vi "Handle Sub Device.vi"(0 "Stand in":refnum<class "Stand.lvclass">, 11 "error in (no error)":errorcluster) -> (4 "Stand out":refnum<class "Stand.lvclass">, 14 "dt PMG":u32, 15 "error out":errorcluster)   [LabVIEW 2019, in "Stand.lvclass"]
uses:
  Stand.lvclass
  Stand.lvclass/Stand.ctl
  PM_Group_class/PM_Group.lvclass/PM_Group.ctl
  PM_Group_class/HandleCmd.vi
  PM_Group_class/private/Handle M24.vi
  PM_Group_class/private/Handle M12.vi
  PM_Group_class/private/Handle M21.vi
  Engine_1DO_2DI_class/UpdateEngine.vi
  PM_Group_class/PM_Group.lvclass
  Valve_2DO_2DI_class/Valve_2DO_2DI.lvclass
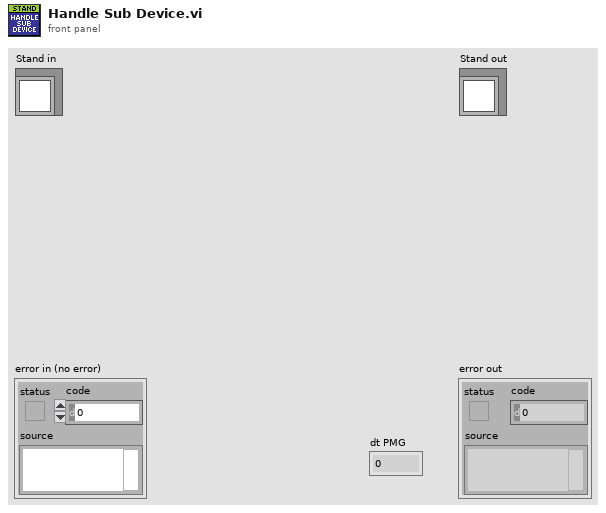
[diagram p1: front panel]
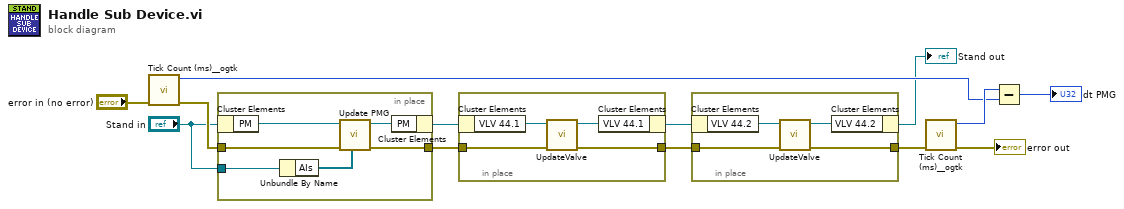
[diagram p0: block diagram]
diagram:
  n1 = call <userlib>:"Tick Count (ms)__ogtk.vi"("error in (no error)"="error in (no error)") -> ("error out"=w12:errorcluster, "millisecond timer value"=w9:u32)  [unwired: 9 in]
  n2 = in-place {
    in-place-border: w12 -> [w17]
    in-place-border: [w14] -> w6
    in-place-border: "Stand in" -> [w16]
    n3 = in-place-cluster #1("Stand in") -> ("PM"=w19:refnum<class "PM_Group.lvclass">)
    n4 = Unbundle By Name(w16) -> ("AIs"=w15:refnum<class "AI.lvclass">[])
    n5 = call "Update PMG.vi"("AIs"=w15, "error in (no error)"=w17, "Pump_1AI_1DO_2DI in"=w19) -> ("error out"=w14:errorcluster, "Pump_1AI_1DO_2DI out"=w18:refnum<class "PM_Group.lvclass">)  [unwired: 7 in]
    n6 = in-place-cluster #1("PM"=w18) -> (w7:refnum<class "Stand.lvclass">)
  }
  n7 = in-place {
    in-place-border: w6 -> [w21]
    in-place-border: [w20] -> w2
    n8 = in-place-cluster #2(w7) -> ("VLV 44.1"=w23:refnum<class "Valve_2DO_2DI.lvclass">)
    n9 = call "UpdateValve.vi"("error in (no error)"=w21, "Pump_1AI_1DO_2DI in"=w23) -> ("error out"=w20:errorcluster, "Pump_1AI_1DO_2DI out"=w22:refnum<class "Valve_2DO_2DI.lvclass">)  [unwired: 8 in]
    n10 = in-place-cluster #2("VLV 44.1"=w22) -> (w5:refnum<class "Stand.lvclass">)
  }
  n11 = in-place {
    in-place-border: [w25] -> w3
    in-place-border: w2 -> [w24]
    n12 = in-place-cluster #3(w5) -> ("VLV 44.2"=w27:refnum<class "Valve_2DO_2DI.lvclass">)
    n13 = call "UpdateValve.vi"("error in (no error)"=w24, "Pump_1AI_1DO_2DI in"=w27) -> ("error out"=w25:errorcluster, "Pump_1AI_1DO_2DI out"=w26:refnum<class "Valve_2DO_2DI.lvclass">)  [unwired: 8 in]
    n14 = in-place-cluster #3("VLV 44.2"=w26) -> (→"Stand out":refnum<class "Stand.lvclass">)
  }
  n15 = call <userlib>:"Tick Count (ms)__ogtk.vi"("error in (no error)"=w3) -> ("error out"=→"error out":errorcluster, "millisecond timer value"=w10:u32)  [unwired: 9 in]
  n16 = Subtract(x=w10, y=w9) -> (x-y=→"dt PMG":u32)
